vi "SecFlow Characteristics.vi"(0 "NDHX Tube Diameter (m)":dbl, 1 "Pipe Diameter (m)":dbl, 2 "Sec Cold Density (kg/m^3)":dbl, 3 "Sec Hot Density (kg/m^3) in":dbl, 4 "Sec Ave Density (kg/m^3) 3":dbl, 5 "FLiNaK Cold Viscosity (Pa-s)":dbl, 6 "FLiNaK Hot Viscosity (Pa-s)":dbl, 8 "Shell Crossflow Area (m^2)":dbl, 9 "FLiNaK Ave Viscosity (Pa-s)":dbl, 10 "Sec Cold Velocity (m/s)":dbl, 11 "MHX Length (m)":dbl, 12 "Sec Hot Velocity (m/s)":dbl, 13 "Sec Loop Height (m)":dbl, 14 "Sec MHX Velocity (m/s)":dbl, 16 "Sec NDHX Velocity (m/s)":dbl) -> (18 "Numeric":dbl, 19 "EA Friction Factor":dbl, 20 "AB Friction Factor":dbl, 21 "AB Reynolds Number":dbl, 22 "BC Friction Factor":dbl, 23 "BC Reynolds Number":dbl, 24 "CEFriction Factor":dbl, 25 "CE Reynolds Number":dbl, 26 "EA Reynolds Number":dbl)   [LabVIEW 2019]
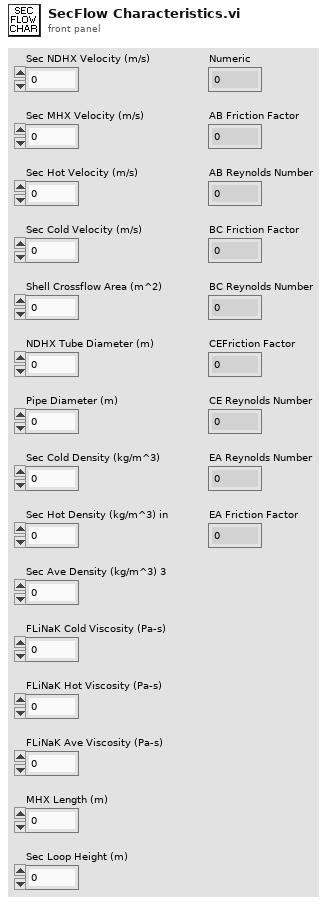
[diagram p1: front panel]
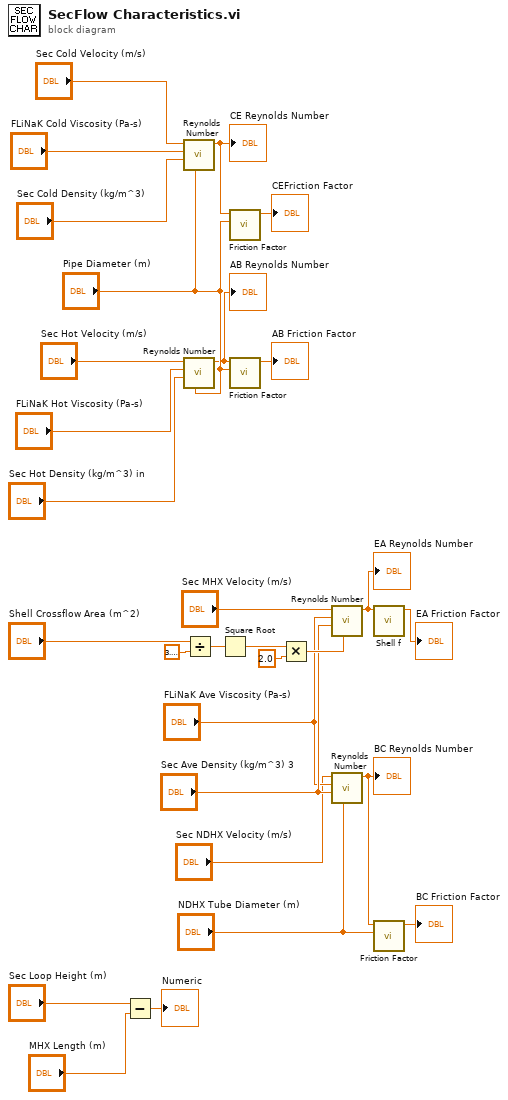
[diagram p0: block diagram]
diagram:
  n1 = Subtract(x="Sec Loop Height (m)", y="MHX Length (m)") -> (x-y=→"Numeric":dbl)
  n2 = call "Reynolds Number.vi"("Effective Length (m)"="Pipe Diameter (m)", "Density (kg/m^3)"="Sec Cold Density (kg/m^3)", "Viscosity (Pa-s)"="FLiNaK Cold Viscosity (Pa-s)", "Velocity (m/s)"="Sec Cold Velocity (m/s)") -> ("Reynolds Number"=w22:dbl)  [unwired: 7 in]
  "CE Reynolds Number" <- w22
  n3 = call "Reynolds Number.vi"("Effective Length (m)"="Pipe Diameter (m)", "Density (kg/m^3)"="Sec Hot Density (kg/m^3) in", "Viscosity (Pa-s)"="FLiNaK Hot Viscosity (Pa-s)", "Velocity (m/s)"="Sec Hot Velocity (m/s)") -> ("Reynolds Number"=w20:dbl)  [unwired: 7 in]
  "AB Reynolds Number" <- w20
  n4 = Divide(x="Shell Crossflow Area (m^2)", y=3.141592653589793) -> (x/y=w16:dbl)
  n5 = Square Root(x=w16) -> (sqrt(x)=w17:dbl)
  n6 = call "Friction Factor.vi"("Effective Length"="Pipe Diameter (m)", "Reynolds Number"=w22) -> ("Friction Factor"=→"CEFriction Factor":dbl)  [unwired: 9 in]
  n7 = call "Friction Factor.vi"("Effective Length"="Pipe Diameter (m)", "Reynolds Number"=w20) -> ("Friction Factor"=→"AB Friction Factor":dbl)  [unwired: 9 in]
  n8 = Multiply(x=w17, y=2.0) -> (x*y=w19:dbl)
  n9 = call "Reynolds Number.vi"("Effective Length (m)"=w19, "Density (kg/m^3)"="Sec Ave Density (kg/m^3) 3", "Viscosity (Pa-s)"="FLiNaK Ave Viscosity (Pa-s)", "Velocity (m/s)"="Sec MHX Velocity (m/s)") -> ("Reynolds Number"=w28:dbl)  [unwired: 7 in]
  "EA Reynolds Number" <- w28
  n10 = call "Reynolds Number.vi"("Effective Length (m)"="NDHX Tube Diameter (m)", "Density (kg/m^3)"="Sec Ave Density (kg/m^3) 3", "Viscosity (Pa-s)"="FLiNaK Ave Viscosity (Pa-s)", "Velocity (m/s)"="Sec NDHX Velocity (m/s)") -> ("Reynolds Number"=w21:dbl)  [unwired: 7 in]
  "BC Reynolds Number" <- w21
  n11 = call "Shell f.vi"("Reynolds Number"=w28) -> ("Numeric"=→"EA Friction Factor":dbl)  [unwired: 10 in]
  n12 = call "Friction Factor.vi"("Effective Length"="NDHX Tube Diameter (m)", "Reynolds Number"=w21) -> ("Friction Factor"=→"BC Friction Factor":dbl)  [unwired: 9 in]
